vi "3.5.1.vi"() -> ()   [LabVIEW 2018]
panel:
  out "출력 클러스터":cluster{"이름":string, "토익 성적":dbl, "성별":bool}
  out "성별 2":bool
  out "토익 성적 2":dbl
  out "이름 2":string
  out "학생":cluster{"이름":string, "토익 성적":dbl, "성별":bool}
  in  "성별":bool
  in  "토익 성적":dbl
  in  "이름":string
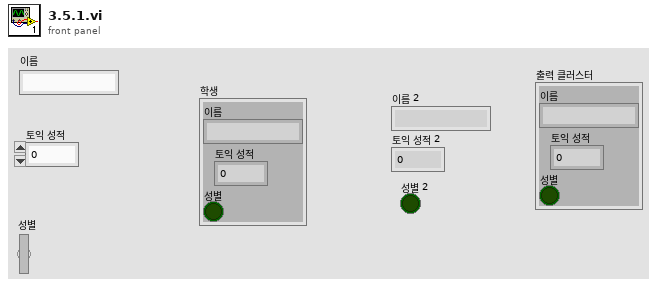
[diagram p1: front panel]
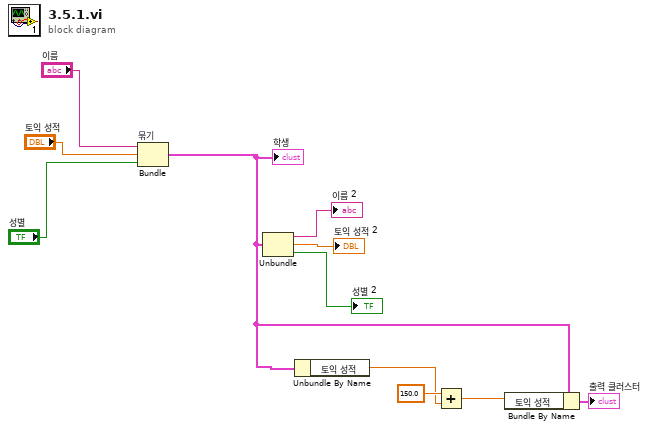
[diagram p0: block diagram]
diagram:
  n1 = Bundle "묶기"("이름"="이름", "토익 성적"="토익 성적", "성별"="성별") -> (w2:cluster{"이름":string, "토익 성적":dbl, "성별":bool})  [unwired: 1 in]
  "학생" <- w2
  n2 = Unbundle(w2) -> ("이름"=→"이름 2":string, "토익 성적"=→"토익 성적 2":dbl, "성별"=→"성별 2":bool)
  n3 = Unbundle By Name(w2) -> ("토익 성적"=w4:dbl)
  n4 = Add(x=150.0, y=w4) -> (x+y=w3:dbl)
  n5 = Bundle By Name(cluster=w2, "토익 성적"=w3) -> (→"출력 클러스터":cluster{"이름":string, "토익 성적":dbl, "성별":bool})
